vi "Test Update JSON Config.vi"() -> ()   [LabVIEW 2019]
uses:
  labview-grpc-query-server/VIs/MeasurementServer_ConfigRequest.ctl
  labview-grpc-query-server/VIs/labview-grpc-measurement-server.lvlib
panel:
  out "output cluster":T1
  in  "ConfigRequest":T1
  in  "JSON Configuration File (.json)":path=path "C:/Users/chericks/Desktop/10_21/Labview-lrms-proof-of-concept/Tesla-LRMS-PoC/jsontestfile.json"
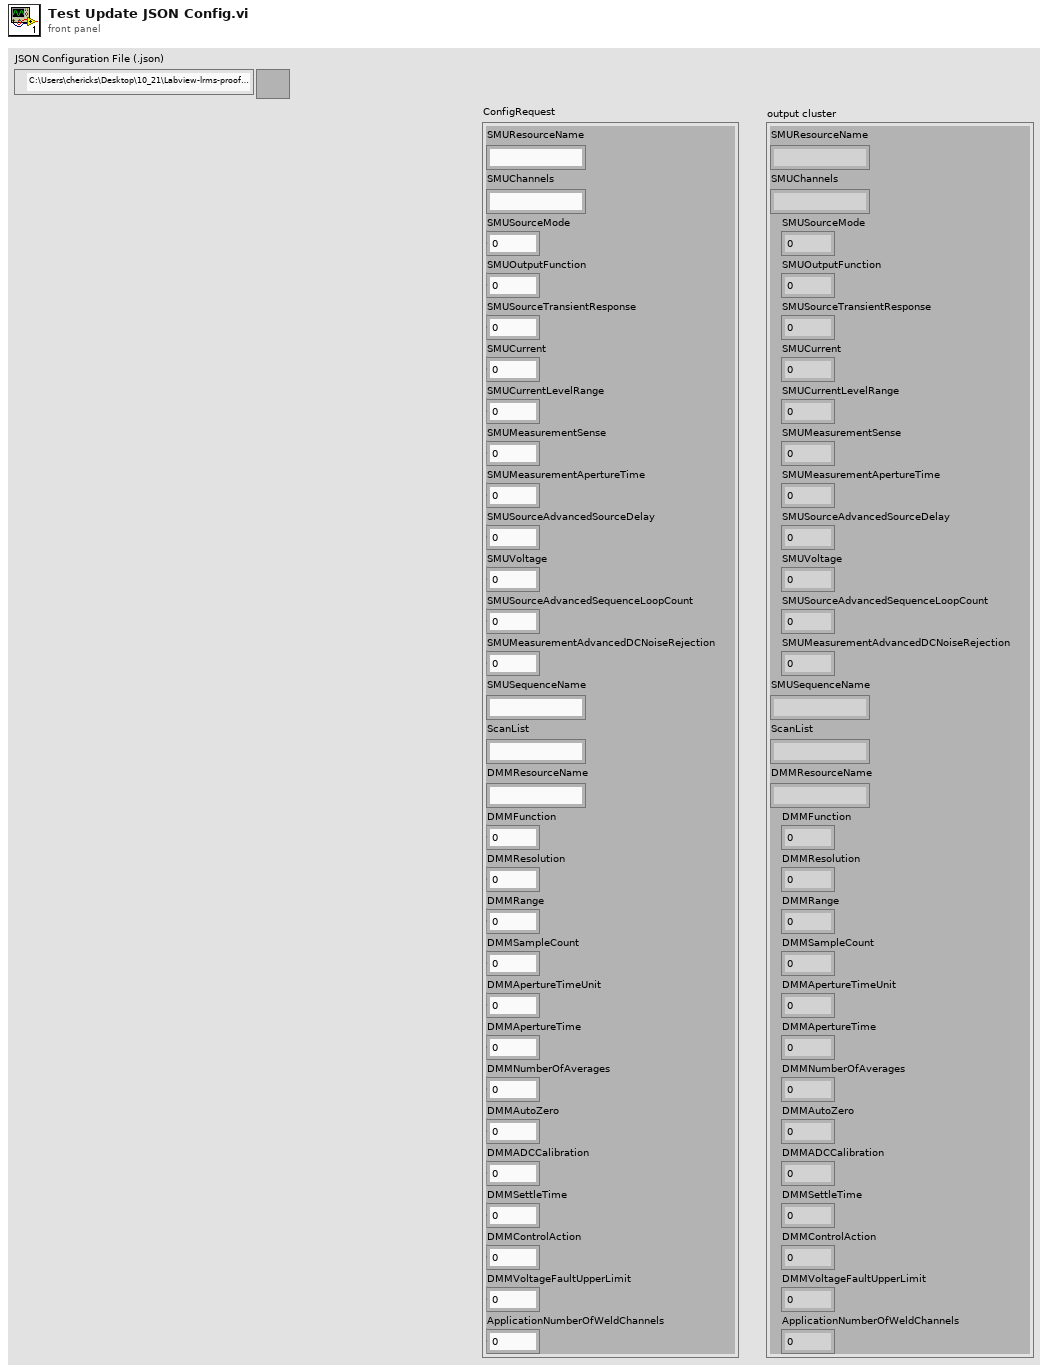
[diagram p1: front panel]
types:
  T1 = typedef "labview-grpc-measurement-server.lvlib/MeasurementServer_ConfigRequest.ctl" = cluster{"SMUResourceName":string, "SMUChannels":string, "SMUSourceMode":i32, "SMUOutputFunction":i32, "SMUSourceTransientResponse":i32, "SMUCurrent":sgl, "SMUCurrentLevelRange":sgl, "SMUMeasurementSense":i32, "SMUMeasurementApertureTime":sgl, "SMUSourceAdvancedSourceDelay":sgl, "SMUVoltage":i32, "SMUSourceAdvancedSequenceLoopCount":i32, "SMUMeasurementAdvancedDCNoiseRejection":i32, "SMUSequenceName":string, "ScanList":string, "DMMResourceName":string, "DMMFunction":i32, "DMMResolution":sgl, "DMMRange":sgl, "DMMSampleCount":i32, "DMMApertureTimeUnit":i32, "DMMApertureTime":sgl, "DMMNumberOfAverages":i32, "DMMAutoZero":i32, "DMMADCCalibration":i32, "DMMSettleTime":sgl, "DMMControlAction":i32, "DMMVoltageFaultUpperLimit":i32, "ApplicationNumberOfWeldChannels":i32}
  T2 = typedef "JSONCluster.ctl" = cluster{"SMUResourceName":string, "SMUChannels":string, "SMUSourceMode":i32, "SMUOutputFunction":i32, "SMUSourceTransientResponse":i32, "SMUCurrent":dbl, "SMUCurrentLevelRange":dbl, "SMUMeasurementSense":i32, "SMUMeasurementApertureTime":dbl, "SMUSourceAdvancedSourceDelay":dbl, "SMUVoltage":dbl, "SMUSourceAdvancedSequenceLoopCount":i32, "SMUMeasurementAdvancedDCNoiseRejection":i32, "SMUSequenceName":string, "SMUStep1_Source_DCCurrent_CurrentLevel":i32, "SMUStep2_Measurement_ApertureTime":i32, "SMUStep3_Source_Advanced_SourceDelay":i32, "SMUSequenceNumberOfSteps":i32, "Switch1ResourceName":string, "Switch1Topology":string, "Switch1ScanList":string, "Switch2ResourceName":string, "Switch2Topology":string, "Switch2ScanList":string, "DMMResourceName":string, "DMMFunction":i32, "DMMResolution":dbl, "DMMRange":dbl, "DMMSampleCount":i32, "DMMApertureTimeUnit":i32, "DMMApertureTime":dbl, "DMMNumberOfAverages":i32, "DMMAutoZero":i32, "DMMADCCalibration":i32, "DMMSettleTime":dbl, "DMMControlAction":i32, "DMMVoltageFaultUpperLimit":dbl, "ApplicationNumberOfWeldChannels":i32}
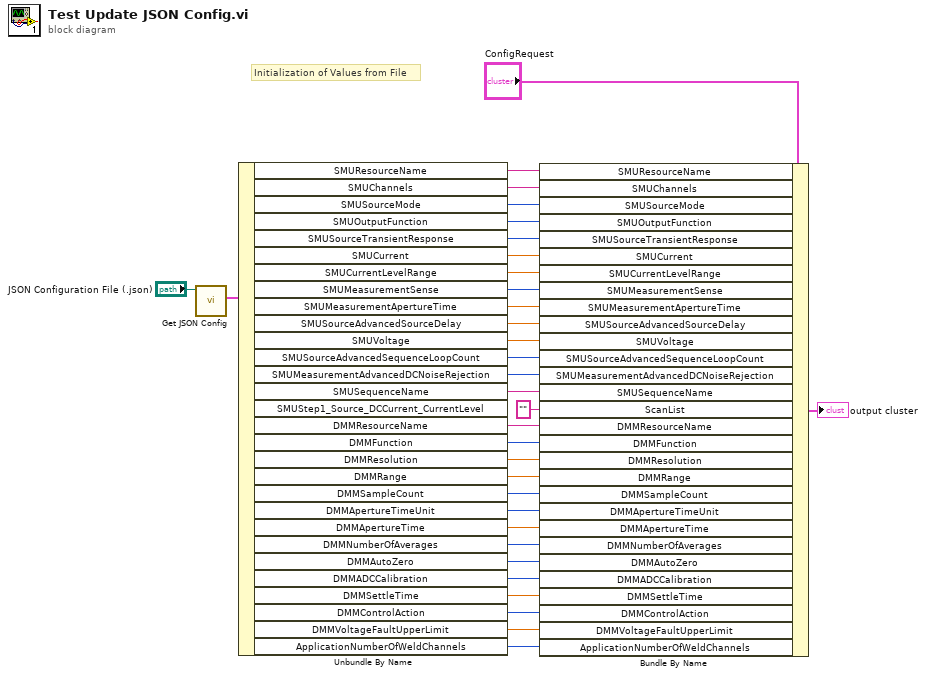
[diagram p0: block diagram]
diagram:
  # "Initialization of Values from File"
  n1 = call "Get JSON Config.vi"("JSON Configuration File (.json)"="JSON Configuration File (.json)") -> ("JSONCluster"=w31:T2)  [unwired: 7 in, 3 out]
  n2 = Unbundle By Name(w31) -> ("SMUResourceName"=w30:string, "SMUChannels"=w29:string, "SMUSourceMode"=w28:i32, "SMUOutputFunction"=w27:i32, "SMUSourceTransientResponse"=w26:i32, "SMUCurrent"=w25:dbl, "SMUCurrentLevelRange"=w24:dbl, "SMUMeasurementSense"=w23:i32, "SMUMeasurementApertureTime"=w22:dbl, "SMUSourceAdvancedSourceDelay"=w21:dbl, "SMUVoltage"=w16:dbl, "SMUSourceAdvancedSequenceLoopCount"=w20:i32, "SMUMeasurementAdvancedDCNoiseRejection"=w19:i32, "SMUSequenceName"=w18:string, "DMMResourceName"=w15:string, "DMMFunction"=w14:i32, "DMMResolution"=w13:dbl, "DMMRange"=w12:dbl, "DMMSampleCount"=w11:i32, "DMMApertureTimeUnit"=w10:i32, "DMMApertureTime"=w9:dbl, "DMMNumberOfAverages"=w8:i32, "DMMAutoZero"=w7:i32, "DMMADCCalibration"=w6:i32, "DMMSettleTime"=w5:dbl, "DMMControlAction"=w4:i32, "DMMVoltageFaultUpperLimit"=w3:dbl, "ApplicationNumberOfWeldChannels"=w2:i32)  [unwired: 1 out]
  n3 = Bundle By Name(cluster="ConfigRequest", "SMUResourceName"=w30, "SMUChannels"=w29, "SMUSourceMode"=w28, "SMUOutputFunction"=w27, "SMUSourceTransientResponse"=w26, "SMUCurrent"=w25, "SMUCurrentLevelRange"=w24, "SMUMeasurementSense"=w23, "SMUMeasurementApertureTime"=w22, "SMUSourceAdvancedSourceDelay"=w21, "SMUVoltage"=w16, "SMUSourceAdvancedSequenceLoopCount"=w20, "SMUMeasurementAdvancedDCNoiseRejection"=w19, "SMUSequenceName"=w18, "ScanList"="", "DMMResourceName"=w15, "DMMFunction"=w14, "DMMResolution"=w13, "DMMRange"=w12, "DMMSampleCount"=w11, "DMMApertureTimeUnit"=w10, "DMMApertureTime"=w9, "DMMNumberOfAverages"=w8, "DMMAutoZero"=w7, "DMMADCCalibration"=w6, "DMMSettleTime"=w5, "DMMControlAction"=w4, "DMMVoltageFaultUpperLimit"=w3, "ApplicationNumberOfWeldChannels"=w2) -> (→"output cluster":T1)
